vi "Activity_9.vi"() -> ()   [LabVIEW 2015]
panel:
  in  "stop":bool
  out "output array":string[](array[string])=["Nombre: dscndcjsd\nsxan xdsc\nmnbsdchjdbc\nC:\\Users\\leser\\Dropbox\\Equipo9\\Class_exercise.vi"]
  out "appended array":string[](array[string])=["Nombre: dscndcjsd\nsxan xdsc\nmnbsdchjdbc\nC:\\Users\\leser\\Dropbox\\Equipo9\\Class_exercise.vi"]
  out "resulting string":string="Nombre: dscndcjsd\nsxan xdsc\nmnbsdchjdbc\nC:\\Users\\leser\\Dropbox\\Equipo9\\Class_exercise.vi"
  in  "Path":path=path "C:/Users/leser/Dropbox/Equipo9/Class_exercise.vi"
  in  "input 3":string="Bermúdez"
  in  "input 2":string="Serrano"
  in  "input 1":string="Luis Esteban"
  in  "initial string":string="Nombre: "
  in  "format string":string="%s\\n%s\\n%s\\n%s"
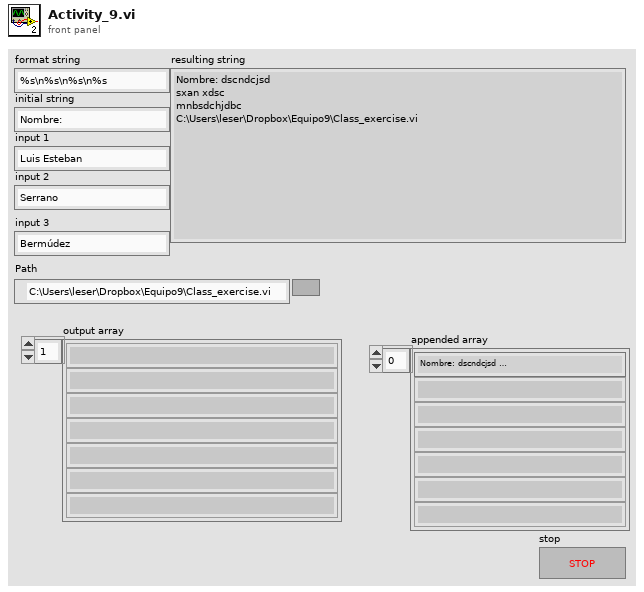
[diagram p1: front panel]
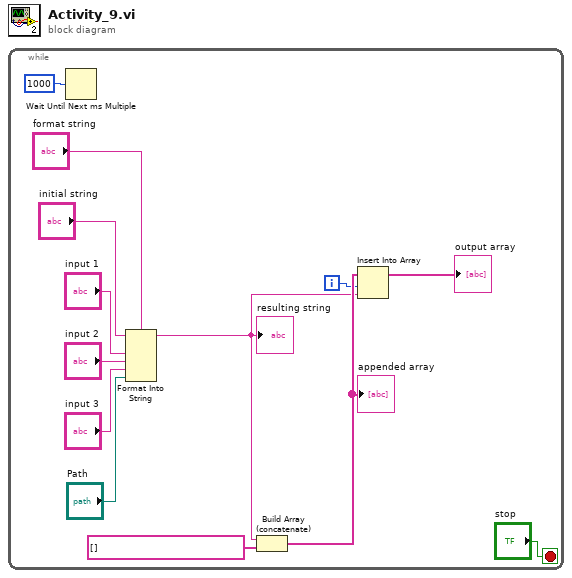
[diagram p0: block diagram]
diagram:
  n1 = while {
    i -> [w5]
    stop <- "stop" stop-if-true
    n2 = Wait Until Next ms Multiple(millisecond multiple=u32 1000) -> ()  [unwired: 1 out]
    n3 = Format Into String "Format Into String"(format string="format string", initial string="initial string", "input 1", "input 2", "input 3", "Path") -> (resulting string=w4:string)  [unwired: 1 in, 1 out]
    "resulting string" <- w4
    n4 = Build Array (concatenate) "Build Array"(w4, string[] []) -> (w6:string[])
    "appended array" <- w6
    n5 = Insert Into Array "Insert Into Array"(array=w6, index=w5, new element=w4) -> (→"output array":string[])
  }
